vi "ApplyLayoutToObject.vi"(5 "scaling settings":T1={"scaling factor"={"horizontal"=1.0, "vertical"=1.0}, "scale text"=FALSE} {"scaling factor"."vertical" min=0.0; "scaling factor"."horizontal" min=0.0}, 7 "properties to ignore":variant, 8 "error in (no error)":errorcluster, 10 "GObj Refnum":refnum<vi>, 11 "Slide Control Layout in":refnum<class "Slide Control Layout.lvclass">) -> (0 "error out":errorcluster, 3 "Slide Control Layout out":refnum<class "Slide Control Layout.lvclass">)   [LabVIEW 2010, in "NI_SE_Front Panel Layout.lvlib" / "Slide Control Layout.lvclass"]
doc: "Apply layout information to the GObj Refnum."
uses:
  Slide Control Layout.lvclass
  NI_SE_Front Panel Layout.lvlib
  NumericWithScale Control Layout/NumericWithScale Control Layout.lvclass
  XY Scaling Factor.ctl
  Scaling Factor_Options.ctl
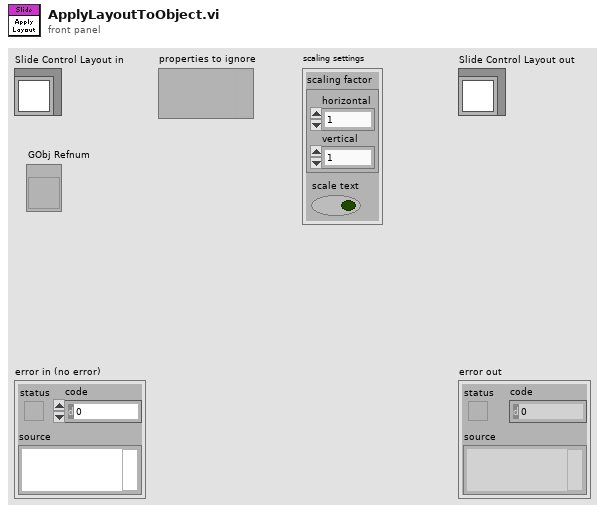
[diagram p1: front panel]
types:
  T1 = typedef "NI_SE_Front Panel Layout.lvlib/Scaling Factor_Options.ctl" = cluster{"scaling factor":T2, "scale text":bool}
  T2 = typedef "NI_SE_Front Panel Layout.lvlib/XY Scaling Factor.ctl" = cluster{"horizontal":dbl, "vertical":dbl}
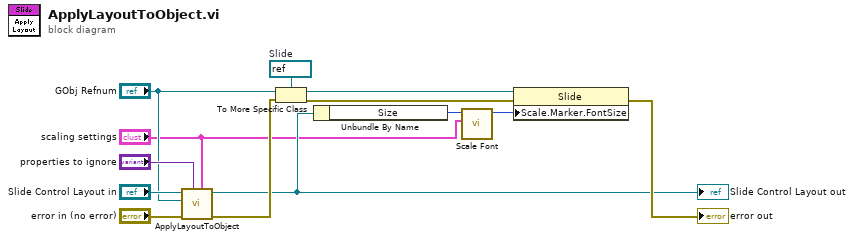
[diagram p0: block diagram]
diagram:
  w5 = refnum<vi> refnum  # Slide
  n1 = call-parent "ApplyLayoutToObject.vi"("scaling settings"="scaling settings", "properties to ignore"="properties to ignore", "error in (no error)"="error in (no error)", "GObj Refnum"="GObj Refnum", "NumericWithScale Control Layout in"="Slide Control Layout in") -> ("error out"=w10:errorcluster, "NumericWithScale Control Layout out"=w7:refnum<class "Slide Control Layout.lvclass">)  [unwired: 5 in]
  "Slide Control Layout out" <- w7
  n2 = To More Specific Class(target class=w5, reference="GObj Refnum", error in=w10) -> (specific class reference=w4:refnum<vi>, error out=w3:errorcluster)
  n3 = Unbundle By Name(w7) -> ("Size"=w2:u16)
  n4 = call "Scale Font.vi"("scaling settings"="scaling settings", "font size in"=w2) -> ("font size out"=w1:u16)  [unwired: 9 in]
  n5 = property class="Slide"(reference=w4, error in=w3, "Scale.Marker.FontSize"=w1) -> (error out=→"error out":errorcluster)  [unwired: 1 out]
